vi "Read Open plot.vi"(8 "error in (no error)":errorcluster, 11 "Pulse Acquired Result in":refnum<class "Pulse Acquired Result.lvclass">) -> (0 "error out":errorcluster, 2 "Open plot":bool, 3 "Pulse Acquired Result out":refnum<class "Pulse Acquired Result.lvclass">)   [LabVIEW 2016, in "Pulse Acquired Result.lvclass"]
uses:
  Pulse Acquired Result.lvclass
  Pulse Acquired Result.lvclass/Pulse Acquired Result.ctl
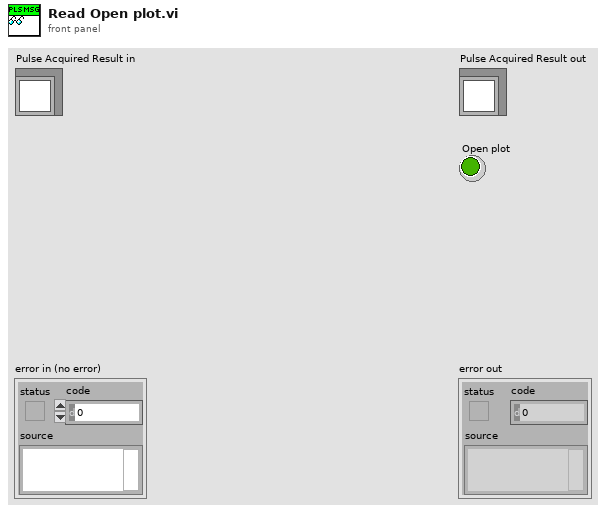
[diagram p1: front panel]
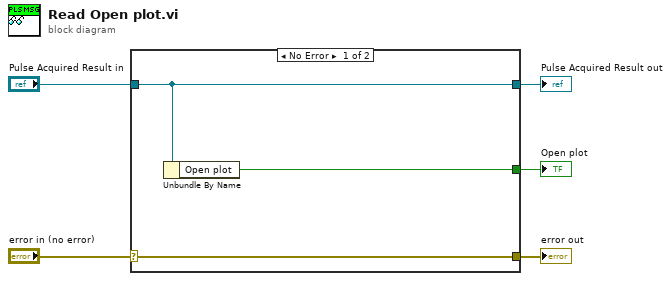
[diagram p0: block diagram]
diagram:
  n1 = case shown="No Error" "error in (no error)" {
    selector: "error in (no error)" -> [w8 w9]
    tunnel: [w8 w9] -> w4
    tunnel: [w7 w10] -> w2
    tunnel: "Pulse Acquired Result in" -> [w7 w10]
    tunnel: [w6 _] -> w1
    frame No Error {
      n2 = Unbundle By Name(w7) -> ("Open plot"=w6:bool)
    }
    frame Error {
    }
  }
  "error out" <- w4
  "Pulse Acquired Result out" <- w2
  "Open plot" <- w1
